vi "Read U32 FIFO - 4x4 spc.vi"(2 "fifo":refnum<k21>, 12 "ready for output":bool=TRUE) -> (4 "output data":u32[](array[numeric]), 10 "output valid":bool)   [LabVIEW 2023]
uses:
  <vilib>/rvi/DataTransferAndStorage/Container/Common/niFpgaContainerExecOnDevCompGetState.vi
  <vilib>/rvi/Emulation/niFpgaSctlEmulationGetInTimedLoop.vi
  <vilib>/rvi/errors/niFpgaSetErrorForExecOnDevCompSimple.vi
  <vilib>/rvi/eio/common/nirviEmuReportErrorAndStop.vi
  <vilib>/rvi/interface/RandomDataEmulation/nirviRandomDataAcquireLock.vi
  <vilib>/rvi/interface/RandomDataEmulation/nirviRandomDataQueueStore.vi
  <vilib>/rvi/interface/RandomDataEmulation/nirviRandomDataReleaseLock.vi
  <vilib>/rvi/interface/RandomDataEmulation/nirviFPGAContextMergeError.vi
  <vilib>/rvi/interface/RandomDataEmulation/nirviRandomDataCheckExitLoopConditions.vi
  <vilib>/express/rvi/timingcommon/nirviCommon.vi
  <vilib>/rvi/interface/RandomDataEmulation/niFpgaRandomDataHandleErrors.vi
  <vilib>/rvi/DataTransferAndStorage/Container/XNode/niFpgaContainer.xnode
  <vilib>/rvi/FIFO/Fifo_Resource/niFpgaFifoEmulationRefInMultiElement.vi
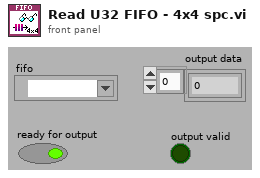
[diagram p1: front panel]
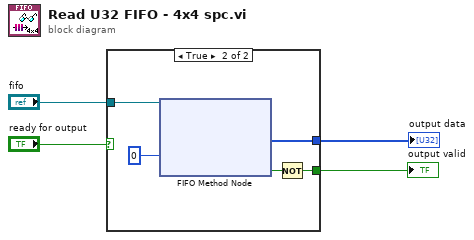
[diagram p0: block diagram]
diagram:
  n1 = case shown="True" "ready for output" {
    tunnel: "fifo" -> [_ w8]
    tunnel: [_ w6] -> w1
    tunnel: [_ w9] -> w3
    frame False {
    }
    frame True {
      n2 = xnode ("FIFO Method Node")("Timeout"=0, "FIFO In"=w8) -> ("Element"=w6:u32[], "Timed Out?"=w5:bool)  [unwired: 1 out]
      n3 = Not(x=w5) -> (.not. x?=w9:bool)
    }
  }
  "output valid" <- w3
  "output data" <- w1
